vi "CoM.vi"(0 "fullfilment consequence":dbl[](array[numeric])=[0.0, 0.25, 0.75] step=0.01 format="%.2f", 1 "consequence":T1(array[cluster])=[{"ling.var."="out", "x-min"=-1.0, "x-max"=1.0, "setarray"=[{"linguistic term"="NEo", "color"=16711680, "points"=[-1.0, -1.0, -1.0, 0.0]}, {"linguistic term"="ZEo", "color"=255, "points"=[-1.0, 0.0, 0.0, 1.0]}, {"linguistic term"="POo", "color"=26214, "points"=[0.0, 1.0, 1.0, 1.0]}]}] {"x-min" format="%.2f"; "x-max" format="%.2f"; "setarray"."points" min=-1.0 max=1.0 step=0.10000000149011612 format="%.2f"}, 2 "active consequence":i32[](array[numeric])=[0, 1, 2], 3 "output when no consequence (0)":u16(ring) items=["last result", "Default"], 4 "output default (0,00)":dbl step=0.009999999776482582 format="%.2f") -> (5 "controller output":dbl step=0.009999999776482582 format="%.2f", 6 "output assessment":string)   [LabVIEW 2017, in "NI_fuzzy logic.lvlib"]
doc: "Defuzzify (Center-of-Maximum) \nThe CoM-Method calculates the prezise outputvalue with the typical values of each fired consequenceterm.\nOutput : Analog value for controlling\nInputs : -consequencearray\n - fullfillment of each term\n - active consequenceterms ...\n - output when no consequence term is firering\n (0: last value , 1: Defaultvalue)\n - output defaultvalue"
uses:
  <vilib>/addons/control/fuzzy/NI_fuzzy logic.lvlib
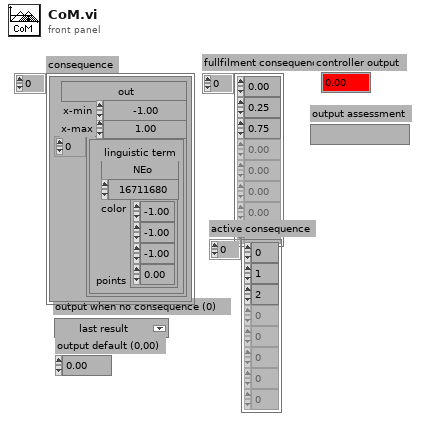
[diagram p1: front panel]
types:
  T1 = cluster{"ling.var.":string, "x-min":dbl, "x-max":dbl, "setarray":cluster{"linguistic term":string, "color":u32, "points":dbl[]}[]}[]
  T2 = cluster{"ling.var.":string, "x-min":dbl, "x-max":dbl, "setarray":cluster{"linguistic term":string, "color":u32, "points":dbl[]}[]}
  T3 = cluster{"linguistic term":string, "color":u32, "points":dbl[]}[]
  T4 = cluster{"linguistic term":string, "color":u32, "points":dbl[]}
  T5 = cluster{"points[0]":dbl, "points[1]":dbl, "points[2]":dbl, "points[3]":dbl}
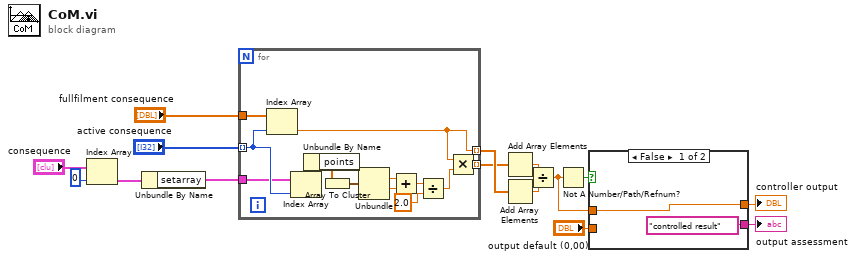
[diagram p0: block diagram]
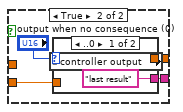
[diagram p2: hidden frame]
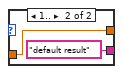
[diagram p3: hidden frame]
diagram:
  n1 = Index Array(array="consequence", index=0) -> (element=w5:T2)
  n2 = Unbundle By Name(w5) -> ("setarray"=w4:T3)
  n3 = for {
    tunnel: "fullfilment consequence" -> [w28]
    tunnel: "active consequence" -> [w27] mode=indexing
    tunnel: [w24] -> w8 mode=indexing
    tunnel: [w25] -> w7 mode=indexing
    tunnel: w4 -> [w23]
    n4 = Index Array(array=w28, index=w27) -> (element=w24:dbl)
    n5 = Index Array(array=w23, index=w27) -> (element=w22:T4)
    n6 = Unbundle By Name(w22) -> ("points"=w21:dbl[])
    n7 = Array To Cluster(array=w21) -> (cluster=w26:T5)
    n8 = Unbundle(w26) -> ("points[1]"=w17:dbl, "points[2]"=w16:dbl)  [unwired: 2 out]
    n9 = Add(x=w17, y=w16) -> (x+y=w18:dbl)
    n10 = Divide(x=w18, y=2.0) -> (x/y=w20:dbl)
    n11 = Multiply(x=w24, y=w20) -> (x*y=w25:dbl)
  }
  n12 = Add Array Elements(numeric array=w7) -> (sum=w12:dbl)
  n13 = Add Array Elements(numeric array=w8) -> (sum=w11:dbl)
  n14 = Divide(x=w12, y=w11) -> (x/y=w9:dbl)
  n15 = Not A Number/Path/Refnum?(number/path/refnum=w9) -> (NaN/Path/Refnum?=w10:bool)
  n16 = case shown="False" w10 {
    tunnel: w9 -> [w30 _]
    tunnel: [w30 w33] -> w2
    tunnel: "output default (0,00)" -> [_ w32]
    tunnel: ["controlled result" w31] -> w1
    frame False {
    }
    frame True {
      n17 = case shown="..0" "output when no consequence (0)" {
        tunnel: [w36 w38] -> w33
        tunnel: w32 -> [_ w38]
        tunnel: ["last result" "default result"] -> w31
        frame ..0 {
          n18 = local read "controller output"() -> (w36:dbl)
        }
        frame 1.. {
        }
      }
    }
  }
  "controller output" <- w2
  "output assessment" <- w1
